vi "WLAN - niVST - RFSG - CommitWaveform.vi"(0 "RFSG handle":refnum<k15>, 5 "RF:Frequency (Hz)":dbl, 7 "RxPower":dbl, 9 "Path Loss":dbl, 11 "WvformNamePostfixed":string, 12 "Number of Packets":i32=50 min=1 max=1000) -> (4 "RFSG handle out":refnum<k15>, 15 "error out":errorcluster)   [LabVIEW 2012]
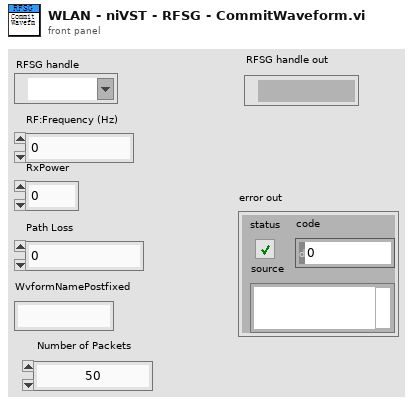
[diagram p1: front panel]
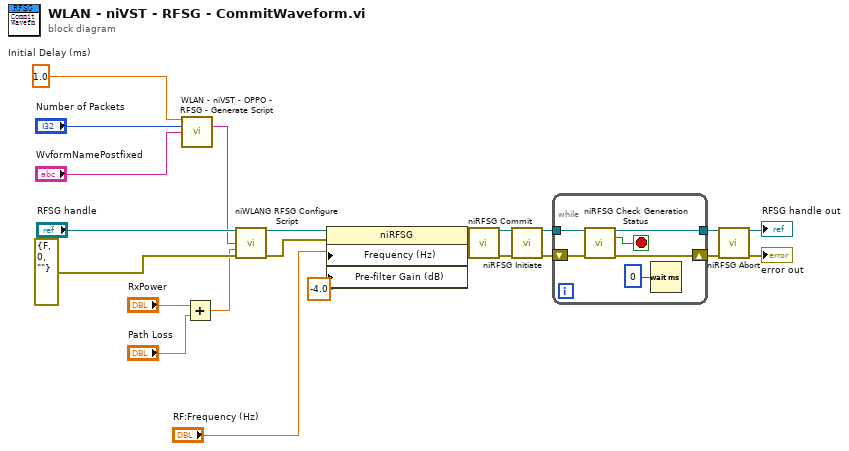
[diagram p0: block diagram]
diagram:
  w13 = 1.0  # Initial Delay (ms)
  n1 = call "WLAN - niVST - OPPO - RFSG - Generate Script.vi"("Initial Delay (ms)"=w13, "Number of Packets"="Number of Packets", "WaveformNamePostfix"="WvformNamePostfixed") -> ("resulting script"=w11:string)  [unwired: 12 in]
  n2 = Add(x="RxPower", y="Path Loss") -> (x+y=w8:dbl)
  n3 = call <vilib>:"niWLANG RFSG Configure Script.vi"("instrument handle"="RFSG handle", "script"=w11, "power level (dBm)"=w8, "error in"=errorcluster {"status"=FALSE, "code"=0, "source"=""} ("error in (no error)")) -> ("instrument handle out"=w7:refnum<k15>, "error out"=w5:errorcluster)  [unwired: 10 in]
  n4 = property class="niRFSG"(reference=w7, error in=w5, "Frequency (Hz)"="RF:Frequency (Hz)", "Pre-filter Gain (dB)"=-4.0 ("Arb:Pre-filter Gain (dB)")) -> (reference out=w6:refnum<k15>, error out=w4:errorcluster)
  n5 = call <instrlib>:"niRFSG Commit.vi"("instrument handle"=w6, "error in"=w4) -> ("instrument handle out"=w19:refnum<k15>, "error out"=w17:errorcluster)  [unwired: 12 in]
  n6 = call <instrlib>:"niRFSG Initiate.vi"("instrument handle"=w19, "error in"=w17) -> ("instrument handle out"=w21:refnum<k15>, "error out"=w18:errorcluster)  [unwired: 12 in]
  n7 = while {
    tunnel: w21 -> [w29]
    tunnel: [w28] -> w20
    shift-right: [w26] -> w16
    shift-left: w18 -> [w25]
    stop <- w27 stop-if-true
    n8 = call <instrlib>:"niRFSG Check Generation Status.vi"("instrument handle"=w29, "error in"=w25) -> ("instrument handle out"=w28:refnum<k15>, "done?"=w27:bool, "error out"=w26:errorcluster)  [unwired: 11 in]
    n9 = Wait (ms)(milliseconds to wait=u32 0) -> ()  [unwired: 1 out]
  }
  n10 = call <instrlib>:"niRFSG Abort.vi"("instrument handle"=w20, "error in"=w16) -> ("instrument handle out"=→"RFSG handle out":refnum<k15>, "error out"=→"error out":errorcluster)  [unwired: 12 in]
